vi "HCC - Fix Ascii.vi"(11 "input string":string) -> (3 "result string":string)   [LabVIEW 2011]
uses:
  Globals HCC.vi
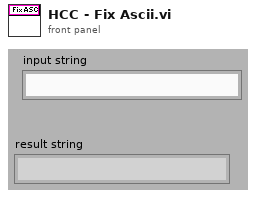
[diagram p1: front panel]
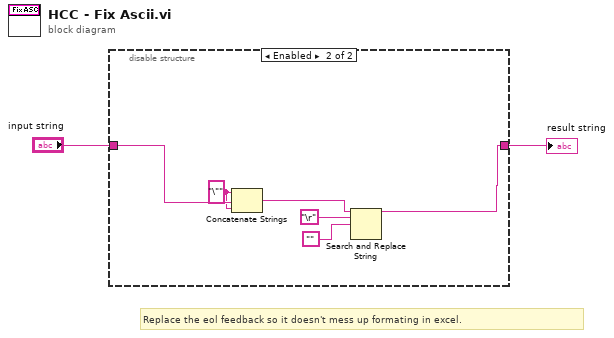
[diagram p0: block diagram]
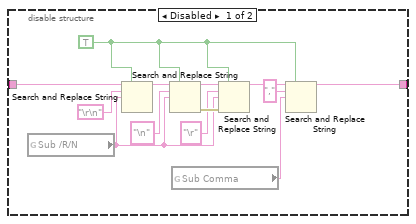
[diagram p2: hidden frame]
diagram:
  # "Replace the eol feedback so it doesn't mess up formating in excel."
  n1 = disable-structure shown="Enabled" {
    disable-tunnel: "input string" -> [w9 w21]
    disable-tunnel: [w4 w16] -> w1
    frame Disabled {
      w3 = TRUE ("replace all? (F)")
      n2 = global read "Globals HCC.vi" "Sub /R/N"() -> (w8:string)
      n3 = Search and Replace String(replace all?=w3, input string=w9, search string="\r\n", replace string=w8) -> (result string=w14:string)  [unwired: 4 in, 3 out]
      n4 = Search and Replace String(replace all?=w3, input string=w14, search string="\n", replace string=w8) -> (result string=w12:string, error out=w11:errorcluster)  [unwired: 4 in, 2 out]
      n5 = global read "Globals HCC.vi" "Sub Comma"() -> (w5:string)
      n6 = Search and Replace String(replace all?=w3, input string=w12, search string="\r", replace string=w8, error in=w11) -> (result string=w7:string)  [unwired: 3 in, 3 out]
      n7 = Search and Replace String(replace all?=w3, input string=w7, search string=",", replace string=w5) -> (result string=w4:string)  [unwired: 4 in, 3 out]
    }
    frame Enabled {
      w20 = "\"" ("string")
      n8 = Concatenate Strings(w20, w21, w20) -> (w17:string)
      n9 = Search and Replace String(input string=w17, search string="\r", replace string="") -> (result string=w16:string)  [unwired: 5 in, 3 out]
    }
  }
  "result string" <- w1
